vi "Measure List Report Status.vi"(8 "error in":errorcluster, 10 "List Number":i32(ring) items=["List 1", "List 2", "List 3", "List 4"], 11 "Instrument Handle In":i32) -> (0 "error out":errorcluster, 1 "Status":u16[](array[numeric]) caption="Measurement Status", 2 "Result":dbl[](array[numeric]), 3 "Instrument Handle Out":i32)   [LabVIEW 8.6, in "ZTScopeM.lvlib"]
doc: "Query the measurement results and status in a measurement list."
uses:
  ZTScopeM.lvlib
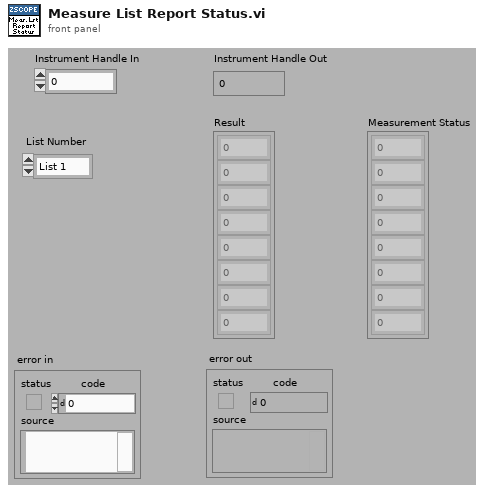
[diagram p1: front panel]
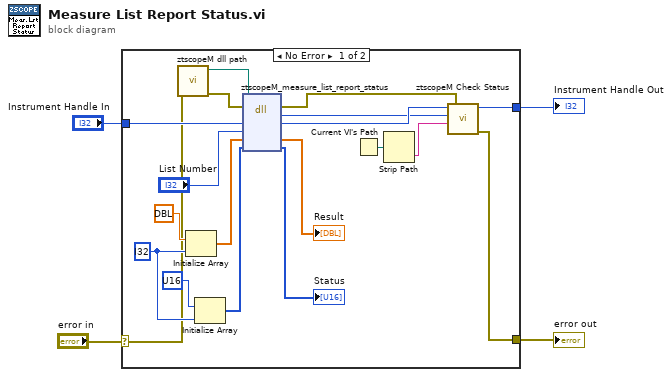
[diagram p0: block diagram]
diagram:
  n1 = case shown="No Error" "error in" {
    selector: "error in" -> [w8 w25]
    tunnel: [w16 w25] -> w1
    tunnel: [w15 w24] -> w4
    tunnel: "Instrument Handle In" -> [w22 w24]
    frame #0 {
      w11 = i32 ? ("dimension size")
      n2 = call "ztscopeM dll path.vi"("error in (no error)"=w8) -> ("error out"=w6:errorcluster, "<instrument>.dll path"=w7:path)  [unwired: 9 in]
      n3 = Initialize Array(dbl ?, w11) -> (w13:dbl[])
      n4 = Initialize Array(u16 ?, w11) -> (w9:u16[])
      n5 = dll-call lib="C:/Program Files (x86)/National Instruments/LabVIEW 2013/instr.lib/ztscopem/ztscopeM.dll" fn="ztscopeM_measure_list_report_status"(path in=w7, error in=w6, "instrumentHandle"=w22, "listNumber"="List Number", "result"=w13, "measurementStatus"=w9) -> (error out=w5:errorcluster, w17:i32, "instrumentHandle"=w18:i32, "result"=→"Result":dbl[], "measurementStatus"=→"Status":u16[])  [unwired: 2 in, 1 out]
      n6 = Current VI's Path() -> (path=w20:path)
      n7 = Strip Path(path=w20) -> (name=w19:string)  [unwired: 1 out]
      n8 = call "ztscopeM Check Status.vi"("error in"=w5, "name of VI"=w19, "status (return code)"=w17, "instrument handle in"=w18) -> ("error out"=w16:errorcluster, "instrument handle out"=w15:i32)  [unwired: 2 in]
    }
    frame #1 {
    }
  }
  "Instrument Handle Out" <- w4
  "error out" <- w1
